vi "Img_Draw_line.vi"(6 "line_width":i32=1, 7 "Color":u32, 8 "error in (no error)":errorcluster, 9 "Point Coordinates 2":cluster{"X":dbl, "Y":dbl}, 10 "Point Coordinates 1":cluster{"X":dbl, "Y":dbl}, 11 "Img In":T1(plugin-control)) -> (0 "error out":errorcluster, 3 "Img out":T1(plugin-control))   [LabVIEW 2021, in "Framework_lib.lvlib"]
uses:
  QMH/Framework_lib.lvlib
  <vilib>/vision/NI_Vision_Development_Module.lvlib
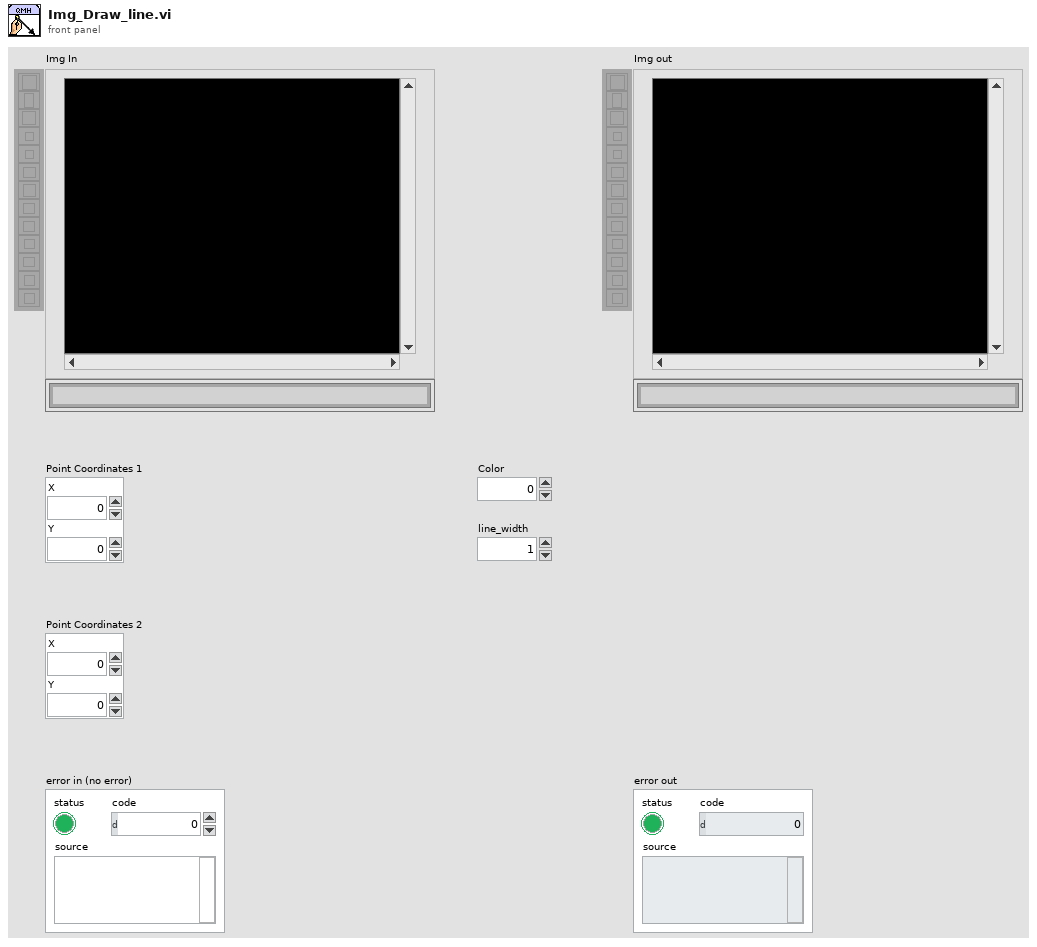
[diagram p1: front panel]
types:
  T1 = typedef "IMAQ Image.ctl" = refnum<image>
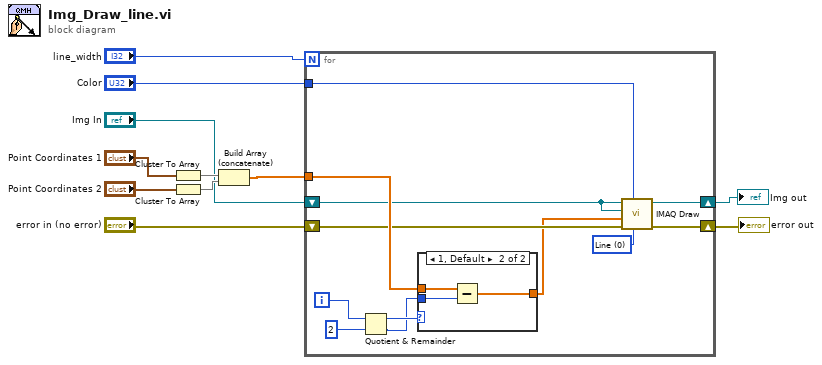
[diagram p0: block diagram]
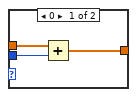
[diagram p2: hidden frame]
diagram:
  n1 = Cluster To Array(cluster="Point Coordinates 1") -> (array=w7:dbl[])
  n2 = Cluster To Array(cluster="Point Coordinates 2") -> (array=w8:dbl[])
  n3 = Build Array (concatenate)(w7, w8) -> (w9:dbl[])
  n4 = for {
    N: "line_width" -> [_]
    tunnel: w9 -> [w23]
    tunnel: "Color" -> [w19]
    shift-right: [w22] -> w6
    shift-left: "error in (no error)" -> [w21]
    shift-right: [w17] -> w2
    shift-left: "Img In" -> [w18]
    i -> [w15]
    w20 = u16 0 items=["Line", "Rectangle", "Oval"] ("Shape to draw")
    n5 = Quotient & Remainder(x=w15, y=2) -> (x-y*floor(x/y)=w13:i32, floor(x/y)=w12:i32)
    n6 = case shown="1, Default" w13 {
      tunnel: w23 -> [w26 w29]
      tunnel: [w25 w28] -> w16
      tunnel: w12 -> [w24 w27]
      frame 0 {
        n7 = Add(x=w26, y=w24) -> (x+y=w25:dbl[])
      }
      frame 1, Default {
        n8 = Subtract(x=w29, y=w27) -> (x-y=w28:dbl[])
      }
    }
    n9 = call "IMAQ Draw"("Shape to draw"=w20, "Pixel Color"=w19, "error in (no error)"=w21, "Coordinates"=w16, "Image Dst"=w18, "Image Src"=w18) -> ("error out"=w22:errorcluster, "Image Dst Out"=w17:T1)  [unwired: 4 in]
  }
  "error out" <- w6
  "Img out" <- w2
